vi "FTW-App-VersionToString.vi"(8 "Build":i32, 9 "Fix":i32, 10 "Minor":i32, 11 "Major":i32) -> (1 "Version (minus Build)":string, 2 "Version String":string)   [LabVIEW 2012]
panel:
  # "Inputs"
  # "Outputs"
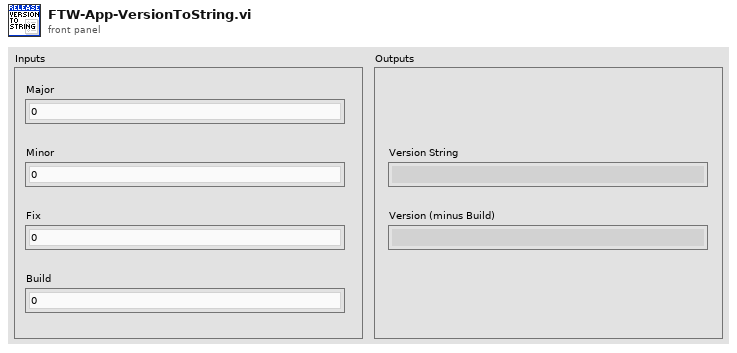
[diagram p1: front panel]
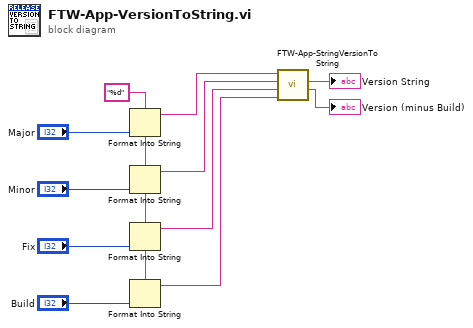
[diagram p0: block diagram]
diagram:
  w1 = "%d" ("format string")
  n1 = Format Into String(format string=w1, "Major") -> (resulting string=w6:string)  [unwired: 2 in, 1 out]
  n2 = Format Into String(format string=w1, "Minor") -> (resulting string=w5:string)  [unwired: 2 in, 1 out]
  n3 = Format Into String(format string=w1, "Fix") -> (resulting string=w4:string)  [unwired: 2 in, 1 out]
  n4 = Format Into String(format string=w1, "Build") -> (resulting string=w3:string)  [unwired: 2 in, 1 out]
  n5 = call "FTW-App-StringVersionToString.vi"("Build"=w3, "Fix"=w4, "Minor"=w5, "Major"=w6) -> ("Version String (minus Build)"=→"Version (minus Build)":string, "Version String"=→"Version String":string)  [unwired: 6 in]
